vi "Edgepoints2Polypoints.vi"(10 "Edgepoints In":cluster{"Row":i32, "Col":i32}[][](array[cluster])) -> (3 "Polyline Out":dbl[][][](array[numeric]))   [LabVIEW 2019]
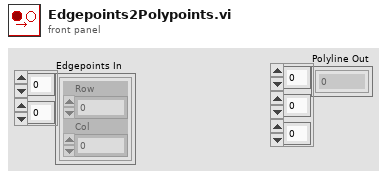
[diagram p1: front panel]
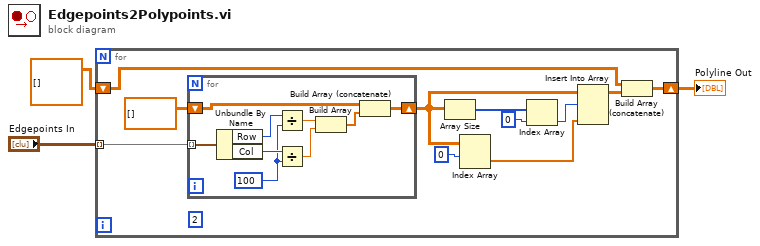
[diagram p0: block diagram]
diagram:
  n1 = for {
    tunnel: "Edgepoints In" -> [w14] mode=indexing
    shift-right: [w13] -> w3
    shift-left: dbl[][][] [] ("Array in") -> [w12]
    (unwired) 2 ("index (row)")
    n2 = for {
      tunnel: w14 -> [w23] mode=indexing
      shift-right: [w22] -> w7
      shift-left: dbl[][] [] -> [w20]
      w15 = 100 ("y")
      n3 = Unbundle By Name(w23) -> ("Row"=w19:i32, "Col"=w18:i32)
      n4 = Divide(x=w19, y=w15) -> (x/y=w17:dbl)
      n5 = Divide(x=w18, y=w15) -> (x/y=w16:dbl)
      n6 = Build Array(w17, w16) -> (w21:dbl[])
      n7 = Build Array (concatenate)(w20, w21) -> (w22:dbl[][])
    }
    n8 = Array Size(array=w7) -> (size(s)=w6:i32[])
    n9 = Index Array(array=w7, index (row)=0) -> (element=w9:dbl[])  [unwired: 1 in]
    n10 = Index Array(array=w6, index=0) -> (element=w4:i32)
    n11 = Insert Into Array(array=w7, index (row)=w4, new element=w9) -> (w8:dbl[][])  [unwired: 1 in]
    n12 = Build Array (concatenate)(w12, w8) -> (w13:dbl[][][])
  }
  "Polyline Out" <- w3
